vi "tx streamer max num samps.vi"(8 "error in (no error)":errorcluster, 10 "max_num_samps_out":u64, 11 "h":u64) -> (0 "error out":errorcluster, 1 "function return":u32(ring), 2 "max_num_samps_out out":u64, 3 "h 2":u64)   [LabVIEW 2024, in "uhd.lvlib"]
doc: "UHD_API uhd_error uhd_tx_streamer_max_num_samps(\n uhd_tx_streamer_handle h, size_t* max_num_samps_out);"
uses:
  uhd.lvlib
  uhd.so
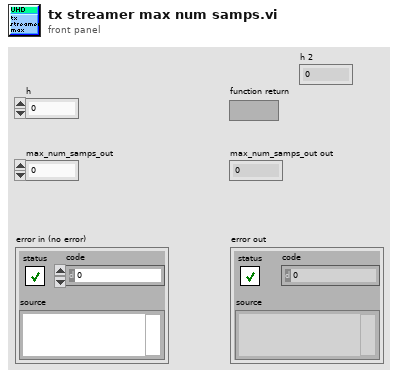
[diagram p1: front panel]
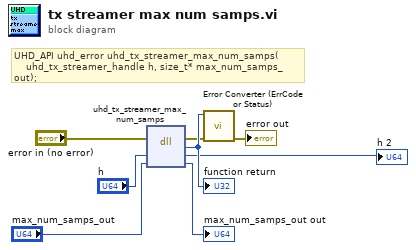
[diagram p0: block diagram]
diagram:
  # "UHD_API uhd_error uhd_tx_streamer_max_num_samps(\n    uhd_tx_streamer_handle h, size_t* max_num_samps_out);"
  n1 = dll-call lib="uhd.*" fn="uhd_tx_streamer_max_num_samps"(error in="error in (no error)", "h"="h", "max_num_samps_out"="max_num_samps_out") -> (error out=w3:errorcluster, w8:u32, "h"=→"h 2":u64, "max_num_samps_out"=→"max_num_samps_out out":u64)  [unwired: 2 in, 1 out]
  "function return" <- w8
  n2 = call "Error Converter (ErrCode or Status).vi"("error in (no error)"=w3, "error code"=w8) -> ("error out"=→"error out":errorcluster)  [unwired: 9 in]
